vi "Get Type.vi"(11 "String 1D in":refnum<class "String 1D.lvclass">) -> (3 "Type":string)   [LabVIEW 2017, in "String 1D.lvclass"]
uses:
  <vilib>/gpm_packages/@cs/data-type-serializer/source/String 1D/String 1D.lvclass
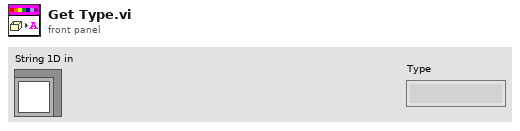
[diagram p1: front panel]
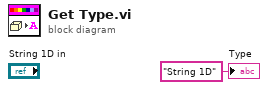
[diagram p0: block diagram]
diagram:
  "Type" <- "String 1D" ("Type")
